vi "Update Result Name.vi"(7 "LabVIEW Result Name Parameter":string="SpecAn Measurement Parameters.Analysis Parameters.Result Name", 8 "error in (no error)":errorcluster, 10 "Step In":refnum<k7>, 11 "SPECAN_IQSLOT in":refnum<class "SPECAN_IQSLOT.lvclass">) -> (0 "error out":errorcluster, 2 "Step Out":refnum<k7>, 3 "SPECAN_IQSLOT out":refnum<class "SPECAN_IQSLOT.lvclass">)   [LabVIEW 2018, in "SPECAN_IQSLOT.lvlib" / "SPECAN_IQSLOT.lvclass"]
uses:
  SPECAN_IQSLOT.lvclass
  C:/Sequence Automation/Plugins/Measurement Interface.lvlibp/Measurement Interface.lvclass
  Plugins/Measurement Interface.lvlibp/Private Methods/Measurement Name/Read Measurement Name.vi
  Plugins/TestStand API Tools (TSAT).lvlibp/Step Actions/TSAT Step Actions.lvlib
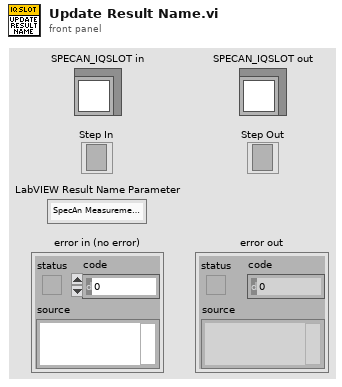
[diagram p1: front panel]
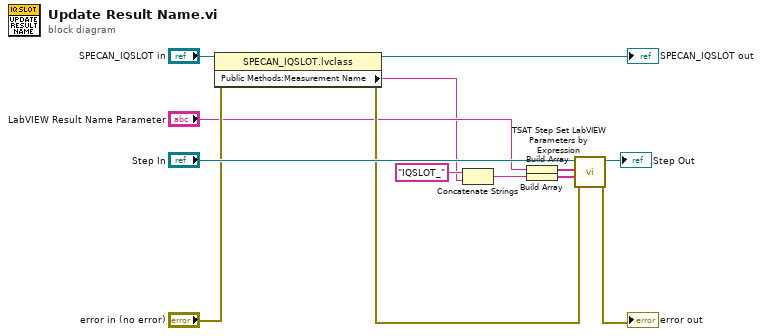
[diagram p0: block diagram]
diagram:
  n1 = property class="SPECAN_IQSLOT.lvclass"(reference="SPECAN_IQSLOT in", error in="error in (no error)") -> (reference out=→"SPECAN_IQSLOT out":refnum<class "SPECAN_IQSLOT.lvclass">, error out=w7:errorcluster, "Public Methods:Measurement Name"=w2:string)
  n2 = Concatenate Strings("IQSLOT_" ("string"), w2) -> (w1:string)
  n3 = Build Array("LabVIEW Result Name Parameter") -> (w11:string[])
  n4 = Build Array(w1) -> (w9:string[])
  n5 = call "TSAT Step Set LabVIEW Parameters by Expression.vi"("Error In"=w7, "Value Expressions"=w9, "Parameters to Set"=w11, "Step In"="Step In") -> ("Error Out"=→"error out":errorcluster, "Step Out"=→"Step Out":refnum<k7>)  [unwired: 6 in]
